vi "IdentifyEG_G_Lockin.vi"(8 "error in (no error)":errorcluster, 11 "VISA Resource Name":refnum<visa-resource-name>) -> (0 "error out":errorcluster, 1 "Identified":bool, 2 "Instrument":T1=enum."LkShr 340 chA&B", 3 "VISA Resource Name Out":refnum<visa-resource-name>)   [LabVIEW 2015]
uses:
  OO Devices/Device/Device type.ctl
  GPIB/VISA  Send Receive.vi
panel:
  out "data":string
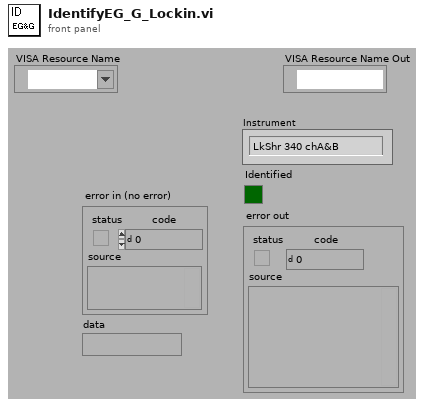
[diagram p1: front panel]
types:
  T1 = typedef "Device type.ctl" = enum16{"NONE", "Neocera 21", "LakeShore 335", "LakeShore 340", "LkShr 340 chA&B", "LakeShore 370", "SRS 850", "SRS 830", "LR 700", "EG&G 5302", "EG&G 7260", "EG&G 7280", "AH 2500", "Keithley meter", "Keithley electrometer", "Keithley 182", "HP 5385", "HP 53181", "HP 53132", "ITC503", "IPS120", "Oxford Mercury IPS", "Oxford PS", "Test", "DC Facility Magnet", "Cryomagnetics PS", "Keithley 2400", "Keithley current source", "Cryo-Con 22C", "HP87NN", "HP4395A"}
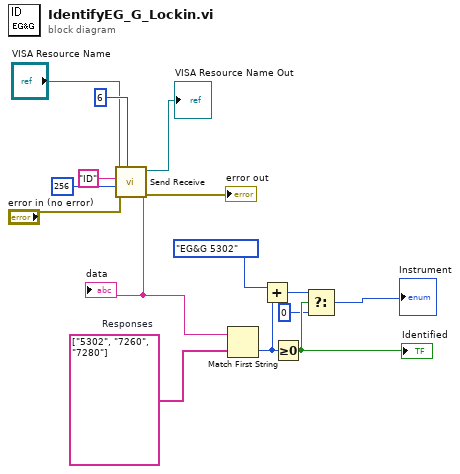
[diagram p0: block diagram]
diagram:
  w13 = string[] ["5302", "7260", "7280"]  # Responses
  n1 = call-poly "Send Receive.vi"("Delay, ms"=u32 6, "error in (no error)"="error in (no error)", "Receive count"=256 ("byte count"), "data string in"="ID", "VISA Resource Name"="VISA Resource Name") -> ("error out"=→"error out":errorcluster, "data string out"=w10:string, "VISA Resource Name Out"=→"VISA Resource Name Out":refnum<visa-resource-name>)  [unwired: 4 in]
  "data" <- w10
  n2 = Match First String(2:w13, 3:w10) -> (0:w11:i32)  [unwired: 1 out]
  n3 = Add(x=Device_type."EG&G 5302", y=w11) -> (x+y=w12:i32)
  n4 = Greater Or Equal To 0?(x=w11) -> (x >= 0?=w14:bool)
  "Identified" <- w14
  n5 = Select(t=w12, s=w14, f=0) -> (s? t:f=→"Instrument":i32)
